vi "Pulse.vi"(10 "Input":bool) -> (2 "Output":bool)   [LabVIEW 2016]
panel:
  # "Sends out  a pulse only on the iteration the Input changes from false to true."
  # "Could be used when you want a joystick action to only happen once."
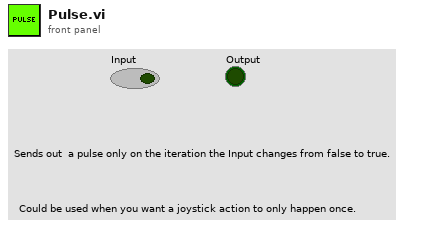
[diagram p1: front panel]
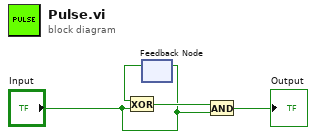
[diagram p0: block diagram]
diagram:
  n1 = feedback-in #1("Input") -> ()
  n2 = feedback #1() -> (w4:bool)  [unwired: 1 in]
  n3 = Exclusive Or(1:"Input", 2:w4) -> (0:w3:bool)
  n4 = And(x=w3, y="Input") -> (x .and. y?=→"Output":bool)
